vi "create new folder.vi"() -> ()   [LabVIEW 2021]
panel:
  in  "Folder Name 2":string
  out "created path 2":path
  out "created path":path
  in  "Folder Name":string
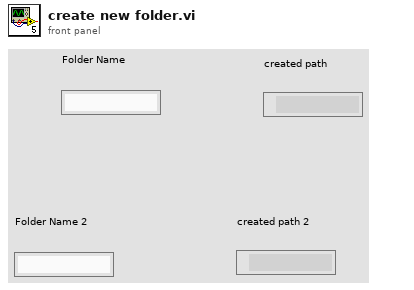
[diagram p1: front panel]
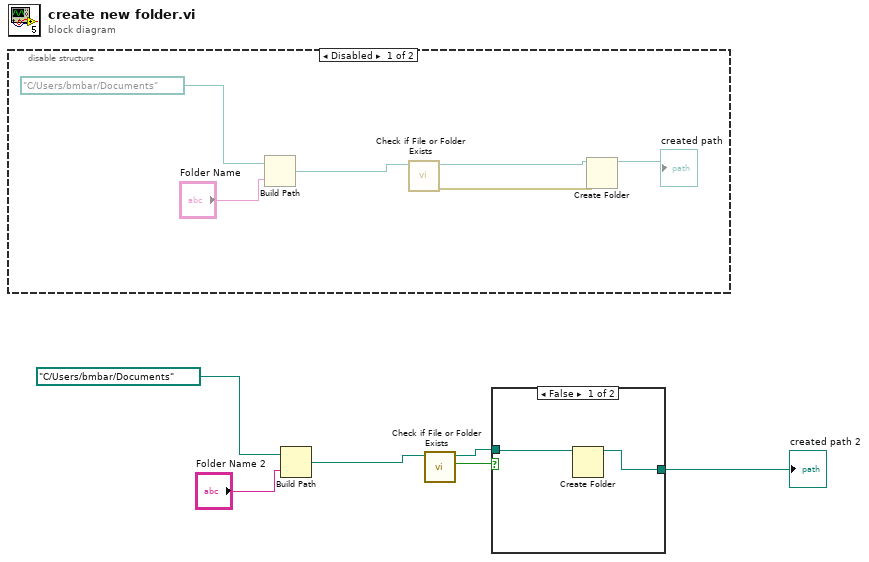
[diagram p0: block diagram]
diagram:
  n1 = disable-structure shown="Disabled" {
    frame Disabled {
      n2 = Build Path(base path=path "C:/Users/bmbar/Documents", name or relative path="Folder Name") -> (appended path=w12:path)
      n3 = call <vilib>:"Check if File or Folder Exists.vi"("path"=w12) -> ("error out"=w7:errorcluster, "dup path"=w11:path)  [unwired: 8 in, 1 out]
      n4 = Create Folder(path (use dialog)=w11, error in=w7) -> (created path=→"created path":path)  [unwired: 1 in, 2 out]
    }
    frame Enabled {
    }
  }
  n5 = Build Path(base path=path "C:/Users/bmbar/Documents", name or relative path="Folder Name 2") -> (appended path=w4:path)
  n6 = call <vilib>:"Check if File or Folder Exists.vi"("path"=w4) -> ("file or folder exists?"=w2:bool, "dup path"=w3:path)  [unwired: 8 in, 1 out]
  n7 = case shown="False" w2 {
    tunnel: w3 -> [w14 w15]
    tunnel: [w13 w15] -> w1
    frame False {
      n8 = Create Folder(path (use dialog)=w14) -> (created path=w13:path)  [unwired: 2 in, 2 out]
    }
    frame True {
    }
  }
  "created path 2" <- w1
